vi "create standard file path.vi"(6 "error in (no error)":errorcluster, 7 "base path":path, 8 "filename":string) -> (0 "error out":errorcluster, 2 "complete\n path":path)   [LabVIEW 2012]
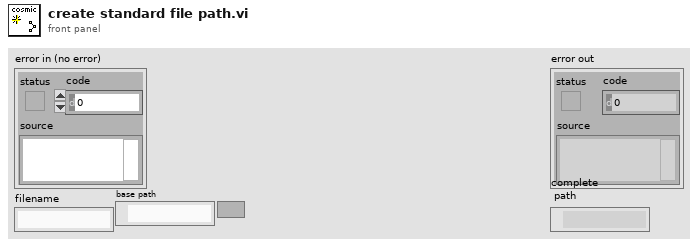
[diagram p1: front panel]
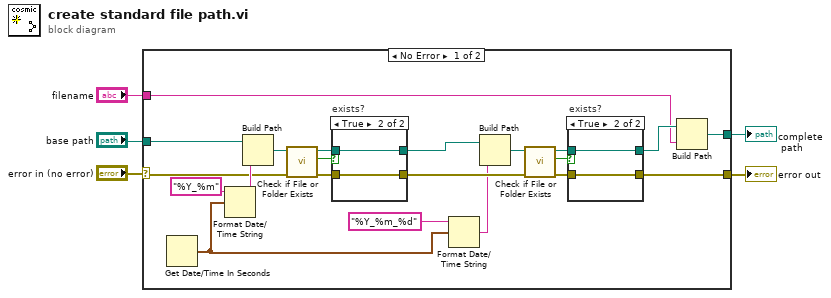
[diagram p0: block diagram]
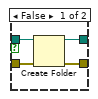
[diagram p2: hidden frame]
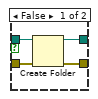
[diagram p3: hidden frame]
diagram:
  n1 = case shown="No Error" "error in (no error)" {
    selector: "error in (no error)" -> [w9 w39]
    tunnel: [w10 w39] -> w4
    tunnel: "filename" -> [w8 _]
    tunnel: [w7 _] -> w2
    tunnel: "base path" -> [w6 _]
    frame No Error {
      n2 = Get Date/Time In Seconds() -> (seconds since 1Jan1904=w25:timestamp)
      n3 = Format Date/Time String(time format string (%c)="%Y_%m", seconds (now)=w25) -> (date/time string=w11:string)  [unwired: 1 in]
      n4 = Build Path(base path=w6, name or relative path=w11) -> (appended path=w13:path)
      n5 = call <vilib>:"Check if File or Folder Exists.vi"("error in (no error)"=w9, "path"=w13) -> ("error out"=w16:errorcluster, "file or folder exists?"=w14:bool, "dup path"=w15:path)  [unwired: 7 in]
      n6 = case "exists?" shown="True" w14 {
        tunnel: w15 -> [w35 w37]
        tunnel: w16 -> [w36 w38]
        tunnel: [w34 w37] -> w24
        tunnel: [w33 w38] -> w23
        frame False {
          n7 = Create Folder(path (use dialog)=w35, error in=w36) -> (created path=w34:path, error out=w33:errorcluster)  [unwired: 1 in, 1 out]
        }
        frame True {
        }
      }
      n8 = Format Date/Time String(time format string (%c)="%Y_%m_%d", seconds (now)=w25) -> (date/time string=w21:string)  [unwired: 1 in]
      n9 = Build Path(base path=w24, name or relative path=w21) -> (appended path=w17:path)
      n10 = call <vilib>:"Check if File or Folder Exists.vi"("error in (no error)"=w23, "path"=w17) -> ("error out"=w20:errorcluster, "file or folder exists?"=w18:bool, "dup path"=w19:path)  [unwired: 7 in]
      n11 = case "exists?" shown="True" w18 {
        tunnel: w19 -> [w29 w31]
        tunnel: w20 -> [w30 w32]
        tunnel: [w28 w31] -> w26
        tunnel: [w27 w32] -> w10
        frame False {
          n12 = Create Folder(path (use dialog)=w29, error in=w30) -> (created path=w28:path, error out=w27:errorcluster)  [unwired: 1 in, 1 out]
        }
        frame True {
        }
      }
      n13 = Build Path(base path=w26, name or relative path=w8) -> (appended path=w7:path)
    }
    frame Error {
    }
  }
  "error out" <- w4
  "complete\n path" <- w2
